vi "Create Single Message.vi"(0 "name":string, 5 "value":string, 7 "attributes":T1, 11 "error in":errorcluster, 12 "priority message (F)":bool, 13 "acknowledge message (F)":bool) -> (4 "message":T2, 15 "error out":errorcluster)   [LabVIEW 2014, in "AMC.lvlib"]
doc: "Creates an AMC message, which can be passed to Send Message.vi."
uses:
  AMC.lvlib
  Message.ctl
  <vilib>/NI/Tools/Keyed Array/KeyedArray.ctl
  <vilib>/NI/Tools/Keyed Array/Tools_KeyedArray.lvlib
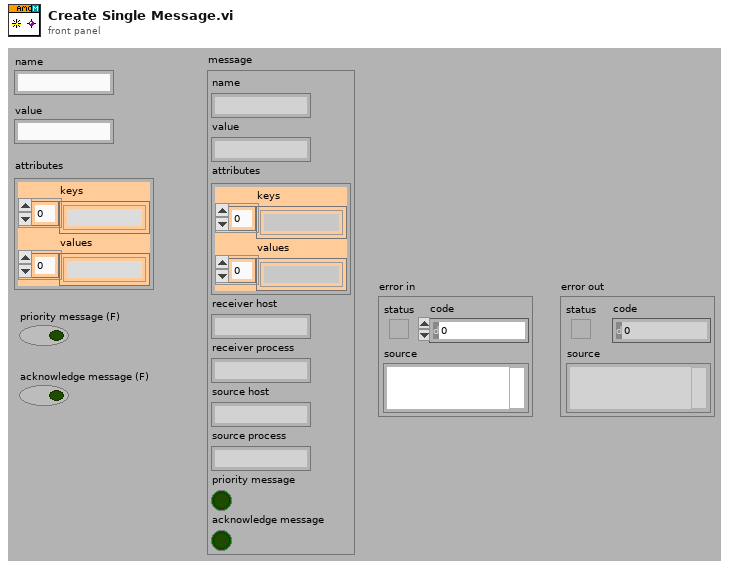
[diagram p1: front panel]
types:
  T1 = typedef "Tools_KeyedArray.lvlib/KeyedArray.ctl" = cluster{"keys":string[], "values":string[]}
  T2 = typedef "AMC.lvlib/Message.ctl" = cluster{"name":string, "value":string, "attributes":T1, "receiver host":string, "receiver process":string, "source host":string, "source process":string, "priority message":bool, "acknowledge message":bool}
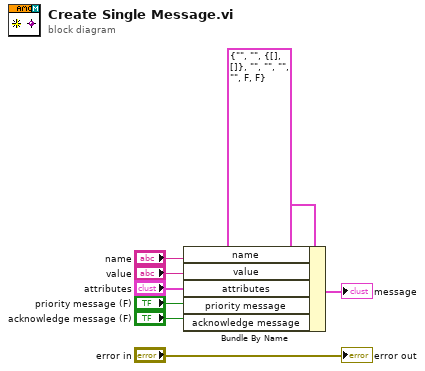
[diagram p0: block diagram]
diagram:
  n1 = Bundle By Name(cluster=T2 {"name"="", "value"="", "attributes"={"keys"=[], "values"=[]}, "receiver host"="", "receiver process"="", "source host"="", "source process"="", "priority message"=FALSE, "acknowledge message"=FALSE} ("Message"), "name"="name", "value"="value", "attributes"="attributes", "priority message"="priority message (F)", "acknowledge message"="acknowledge message (F)") -> (→"message":T2)
  "error out" <- "error in"
